vi "Label Targets3.vi"(7 "Annotate":bool=TRUE, 8 "Score Threshold":dbl, 9 "results":T1, 11 "Image in":T2) -> (3 "Image out":T2)   [LabVIEW 2019]
doc: "Draw scores near or on the particle and an ellipse around the target. Scores that are below the score threshold are drawn in red, above in green."
uses:
  <vilib>/vision/Image Controls.llb/IMAQ Image.ctl
  Target Fields.ctl
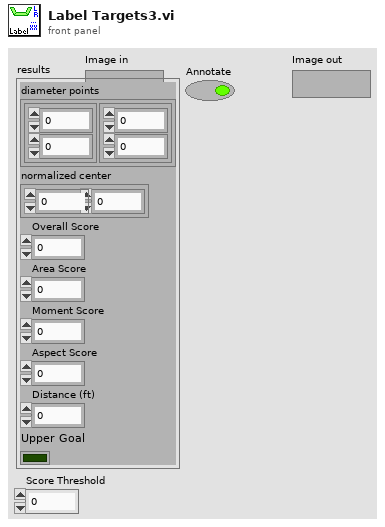
[diagram p1: front panel]
types:
  T1 = typedef "Target Fields.ctl" = cluster{"diameter points":cluster{"first point":cluster{"x":dbl, "y":dbl}, "projected point":cluster{"x":dbl, "y":dbl}}, "normalized center":cluster{"x":dbl, "y":dbl}, "Overall Score":dbl, "Area Score":dbl, "Moment Score":dbl, "Aspect Score":dbl, "Distance (ft)":dbl, "Upper Goal":bool}
  T2 = typedef "IMAQ Image.ctl" = refnum<image>
  T3 = cluster{"Desired Font (Application)":enum16{"User-specified Font", "Application Font", "System Font", "Dialog Font"}, "[User-specified Font]":cluster{"Font Name":string, "Size":i16, "Strikeout?":bool, "Italic?":bool, "Underline?":bool, "Outline?":bool, "Shadow?":bool, "Bold?":bool, "Rotation Angle":dbl}, "Horizontal Alignment":i16, "Vertical Alignment":i16}
  T4 = cluster{"first point":cluster{"x":dbl, "y":dbl}, "projected point":cluster{"x":dbl, "y":dbl}}
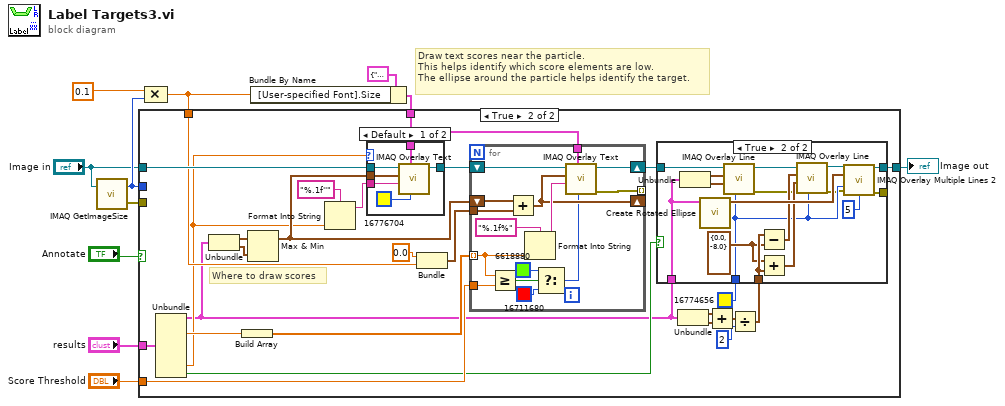
[diagram p0: block diagram]
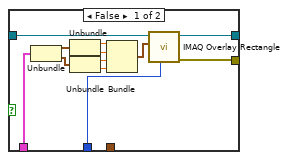
[diagram p3: hidden frame]
diagram:
  # "Draw text scores near the particle.\nThis helps identify which score elements are low.\nThe ellipse around the particle helps identify the target."
  n1 = call "IMAQ GetImageSize"("Image"="Image in") -> ("Y Resolution"=w8:i32, "error out"=w1:errorcluster)  [unwired: 3 in, 1 out]
  n2 = Compound Arithmetic op=MULTIPLY(0.1, w8) -> (w5:dbl)
  n3 = Bundle By Name(cluster=T3 {"Desired Font (Application)"=enum."User-specified Font", "[User-specified Font]"={"Font Name"="Ariel", "Size"=12, "Strikeout?"=FALSE, "Italic?"=FALSE, "Underline?"=FALSE, "Outline?"=FALSE, "Shadow?"=FALSE, "Bold?"=FALSE, "Rotation Angle"=0.0}, "Horizontal Alignment"=0, "Vertical Alignment"=0} ("Font, Size & Style"), "[User-specified Font].Size"=w5) -> (w6:T3)
  n4 = case shown="True" "Annotate" {
    tunnel: [w12 w32] -> w11
    tunnel: "Image in" -> [w12 w38]
    tunnel: w6 -> [_ w21]
    tunnel: w8 -> [_ _]
    tunnel: w5 -> [_ w34]
    tunnel: "results" -> [_ w33]
    tunnel: "Score Threshold" -> [_ w23]
    tunnel: w1 -> [_ _]
    frame False {
    }
    frame True {
      # "Where to draw scores"
      n5 = Unbundle(w33) -> ("diameter points"=w18:T4, "Overall Score"=w31:dbl, "Distance (ft)"=w22:dbl, "Upper Goal"=w20:bool)  [unwired: 4 out]
      n6 = Unbundle(w18) -> ("first point"=w25:cluster{"x":dbl, "y":dbl}, "projected point"=w26:cluster{"x":dbl, "y":dbl})
      n7 = Build Array(w31) -> (w28:dbl[])
      n8 = Max & Min(x=w25, y=w26) -> (max(x,y)=w24:cluster{"x":dbl, "y":dbl})  [unwired: 1 out]
      n9 = Format Into String(format string="%.1f''", w22) -> (resulting string=w37:string)  [unwired: 2 in, 1 out]
      n10 = case shown="Default" w22 {
        tunnel: w38 -> [w88 w89]
        tunnel: w37 -> [w87 _]
        tunnel: w21 -> [w86 _]
        tunnel: [w85 w89] -> w30
        tunnel: w24 -> [w84 _]
        frame Default {
          n11 = call "IMAQ Overlay Text"("Text Color (black)"=u32 16776704 ("Color"), "Font, Size & Style"=w86, "String"=w87, "Origin"=w84, "Image"=w88) -> ("Image Out"=w85:T2)  [unwired: 5 in, 1 out]
        }
        frame 0 {
        }
      }
      n12 = Bundle(0.0, w34) -> (w27:cluster{dbl, dbl})  [unwired: 1 in]
      n13 = for {
        tunnel: w28 -> [w71] mode=indexing
        shift-right: [w79] -> w29
        shift-left: w30 -> [w80]
        tunnel: w21 -> [w78]
        shift-right: [w75] -> _
        shift-left: w24 -> [w76]
        tunnel: w27 -> [w77]
        tunnel: w23 -> [w70]
        tunnel: [w68] -> _ mode=indexing
        n14 = Greater Or Equal?(x=w71, y=w70) -> (x >= y?=w69:bool)
        n15 = Add(x=w76, y=w77) -> (x+y=w75:cluster{dbl, dbl})
        n16 = Format Into String(format string="%.1f%", w71) -> (resulting string=w81:string)  [unwired: 2 in, 1 out]
        n17 = Select(t=u32 6618880 ("Color"), s=w69, f=u32 16711680 ("Color")) -> (s? t:f=w72:u32)
        n18 = call "IMAQ Overlay Text"("Text Color (black)"=w72, "Font, Size & Style"=w78, "String"=w81, "Origin"=w75, "Image"=w80) -> ("error out"=w68:errorcluster, "Image Out"=w79:T2)  [unwired: 5 in]
      }
      n19 = Unbundle(w18) -> ("first point"=w17:cluster{"x":dbl, "y":dbl}, "projected point"=w16:cluster{"x":dbl, "y":dbl})
      n20 = Add(x=w17, y=w16) -> (x+y=w15:cluster{"x":dbl, "y":dbl})
      n21 = Divide(x=w15, y=u32 2 ("Width")) -> (x/y=w13:cluster{"x":dbl, "y":dbl})
      n22 = case shown="True" w20 {
        tunnel: [w49 w65] -> w32
        tunnel: w18 -> [w47 w62]
        tunnel: w29 -> [w50 w61]
        tunnel: u32 16774656 ("Color") -> [w48 w54]
        tunnel: w13 -> [_ w58]
        tunnel: [w39 w51] -> _
        frame False {
          n23 = Unbundle(w47) -> ("first point"=w46:cluster{"x":dbl, "y":dbl}, "projected point"=w45:cluster{"x":dbl, "y":dbl})
          n24 = Unbundle(w46) -> ("x"=w44:dbl, "y"=w43:dbl)
          n25 = Unbundle(w45) -> ("x"=w42:dbl, "y"=w41:dbl)
          n26 = Bundle("x"=w44, "y"=w43, "x"=w42, "y"=w41) -> (w40:cluster{"x":dbl, "y":dbl, "x":dbl, "y":dbl})  [unwired: 1 in]
          n27 = call "IMAQ Overlay Rectangle"("Color"=w48, "Rectangle"=w40, "Image"=w50) -> ("error out"=w39:errorcluster, "Image Out"=w49:T2)  [unwired: 7 in]
        }
        frame True {
          w55 = cluster{"x":dbl, "y":dbl} {"x"=0.0, "y"=-8.0} ("x/y")
          n28 = Unbundle(w62) -> ("first point"=w67:cluster{"x":dbl, "y":dbl}, "projected point"=w66:cluster{"x":dbl, "y":dbl})
          n29 = call "Create Rotated Ellipse.vi"("diameter points"=w62) -> ("XY Graph"=w64:cluster{"X":dbl, "Y":dbl}[])  [unwired: 10 in]
          n30 = call "IMAQ Overlay Line"("Color"=w54, "End Point"=w66, "Start Point"=w67, "Image"=w61) -> ("error out"=w53:errorcluster, "Image Out"=w60:T2)  [unwired: 6 in]
          n31 = Subtract(x=w58, y=w55) -> (x-y=w57:cluster{"x":dbl, "y":dbl})
          n32 = Add(x=w55, y=w58) -> (x+y=w56:cluster{"x":dbl, "y":dbl})
          n33 = call "IMAQ Overlay Line"("Color"=w54, "error in (no error)"=w53, "End Point"=w56, "Start Point"=w57, "Image"=w60) -> ("error out"=w52:errorcluster, "Image Out"=w59:T2)  [unwired: 5 in]
          n34 = call "IMAQ Overlay Multiple Lines 2"("Image"=w59, "Line End Points"=w64, "Color"=w54, "error in (no error)"=w52, "Width"=u32 5) -> ("Image Out"=w65:T2, "error out"=w51:errorcluster)  [unwired: 9 in]
        }
      }
    }
  }
  "Image out" <- w11
